vi "GyroLastValue.vi"() -> ()   [LabVIEW 2015]
panel:
  in  "GyroLastValue":dbl
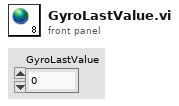
[diagram p1: front panel]
diagram:
